vi "Local Endpoint B2.vi"() -> ()   [LabVIEW 2020]
uses:
  Communication/IP_Communication/typedefs/General Settings.ctl
  Communication/IP_Communication/typedefs/Endpoint Tag.ctl
  Communication/Local/Local.lvclass
  C:/Users/dihidalg/Documents/GitHub/lvoop_exercise1/Exercise Files/Communication/IP_Communication/IP_Communication.lvclass
  Communication/Network/Network.lvclass
  Communication/Packet/Packet.lvclass
  Communication/IP_Communication/IP_Communication.lvclass/IP_Communication.ctl
  Communication/Packet/Packet.lvclass/Packet.ctl
  Communication/IP_Communication/IP_Communication.lvclass
panel:
  in  "General Settings":T1={"Connection Name"="Local_Test", "Endpoint Tag"=enum."B"}
  in  "Local?":bool=TRUE
  in  "Stop VI":bool
  in  "Send Command":bool
  in  "Command ID":u16
  out "Command Rx":T3
  out "Timeout?":bool
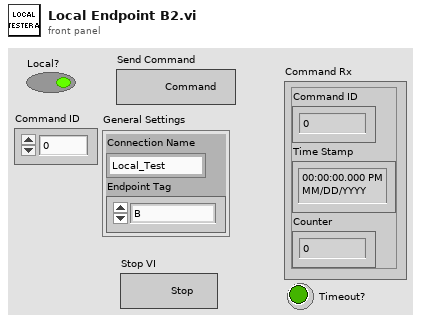
[diagram p1: front panel]
types:
  T1 = typedef "Communication Classes.lvlib/IP_Communication.lvclass/General Settings.ctl" = cluster{"Connection Name":string, "Endpoint Tag":T2}
  T2 = typedef "Communication Classes.lvlib/IP_Communication.lvclass/Endpoint Tag.ctl" = enum8{"A", "B"}
  T3 = cluster{"Command ID":u16, "Time Stamp":timestamp, "Counter":u16}
  T4 = cluster{"Command Out":cluster{"Command ID":u16, "Time Stamp":timestamp, "Counter":u16}, " Timeout?":bool}
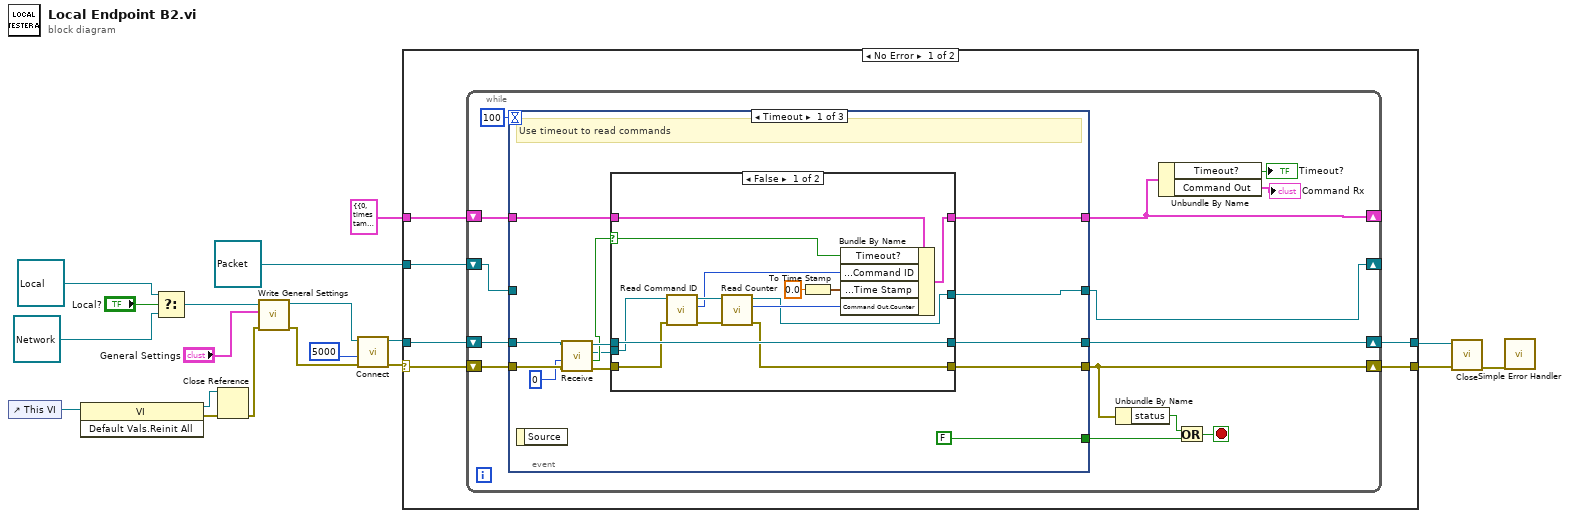
[diagram p0: block diagram]
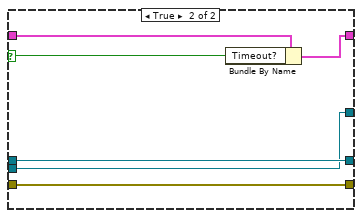
[diagram p2: hidden frame]
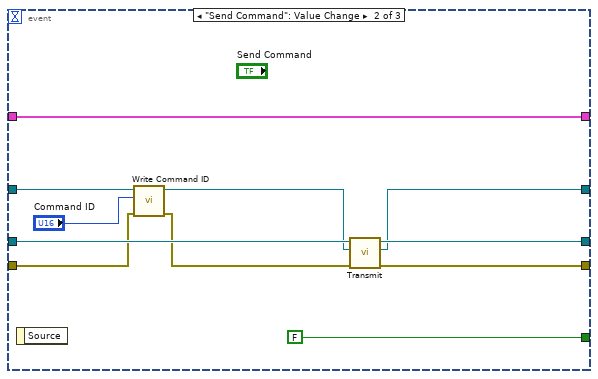
[diagram p3: hidden frame]
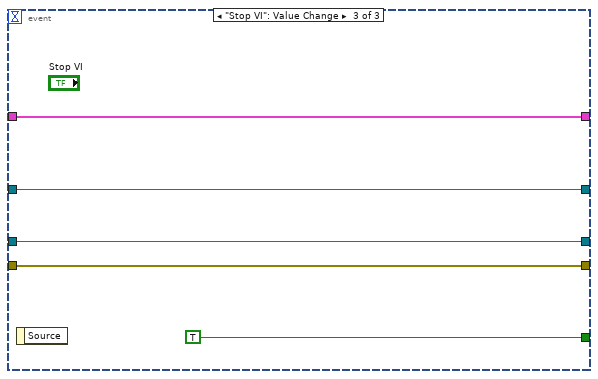
[diagram p4: hidden frame]
diagram:
  n1 = control-ref of="This VI"() -> (w19:refnum<vi>)
  n2 = invoke class="VI" method="Default Vals.Reinit All"(reference=w19) -> (reference out=w17:refnum<vi>, error out=w18:errorcluster)  [unwired: 2 in, 1 out]
  n3 = Select(t=refnum<class "Local.lvclass"> refnum ("Communication Classes.lvlib:Local.lvclass"), s="Local?", f=refnum<class "Network.lvclass"> refnum ("Communication Classes.lvlib:Network.lvclass")) -> (s? t:f=w5:refnum<class "IP_Communication.lvclass">)
  n4 = Close Reference(reference=w17, error in (no error)=w18) -> (error out=w3:errorcluster)
  n5 = call "Write General Settings.vi"("error in (no error)"=w3, "General Settings"="General Settings", "IP_Communication in"=w5) -> ("error out"=w2:errorcluster, "IP_Communication out"=w4:refnum<class "IP_Communication.lvclass">)  [unwired: 7 in]
  n6 = call-dynamic "Connect.vi"("error in (no error)"=w2, "timeout in ms (10000)"=5000 ("Timeout"), "Communication in"=w4) -> ("error out"=w13:errorcluster, "Communication out"=w12:refnum<class "IP_Communication.lvclass">)  [unwired: 7 in]
  n7 = case shown="No Error" w13 {
    selector: w13 -> [w21 w90]
    tunnel: [w23 w90] -> w10
    tunnel: [w22 w89] -> w8
    tunnel: w12 -> [w25 w89]
    tunnel: T4 {"Command Out"={"Command ID"=0, "Time Stamp"=timestamp(0 s since 1904-01-01), "Counter"=0}, " Timeout?"=FALSE} -> [w24 _]
    tunnel: refnum<class "Packet.lvclass"> refnum ("Communication Classes.lvlib:Packet.lvclass") -> [w20 _]
    frame No Error {
      n8 = while {
        shift-right: [w27] -> _
        shift-left: w24 -> [w38]
        shift-right: [w31] -> w22
        shift-left: w25 -> [w37]
        shift-right: [w35] -> w23
        shift-left: w21 -> [w36]
        shift-right: [w29] -> _
        shift-left: w20 -> [w30]
        stop <- w34 stop-if-true
        n9 = event shown="[0] Timeout" {
          selector: _ -> [_ _ _]
          dyn-events: _ -> [_ _ _]
          timeout: 100 -> [_ _ _]
          tunnel: w38 -> [w50 w83 w88]
          tunnel: [w49 w83 w88] -> w27
          tunnel: w37 -> [w48 w81 w84]
          tunnel: w36 -> [w47 w75 w87]
          tunnel: [w52 w78 w87] -> w35
          tunnel: [FALSE FALSE TRUE] -> w32
          tunnel: [w41 w76 w84] -> w31
          tunnel: w30 -> [_ w77 w85]
          tunnel: [w40 w73 w85] -> w29
          event Timeout {
            # "Use timeout to read commands"
            n10 = event-data() -> ()  [unwired: 1 in, 1 out]
            n11 = call-dynamic "Receive.vi"("error in (no error)"=w47, "timeout in ms (0)"=0 ("timeout in ms (-1)"), "Communication in"=w48) -> ("error out"=w43:errorcluster, "Timeout?"=w44:bool, "Packet Received"=w42:refnum<class "Packet.lvclass">, "Communication out"=w45:refnum<class "IP_Communication.lvclass">)  [unwired: 5 in]
            n12 = case shown="False" w44 {
              selector: w44 -> [w64 w69]
              tunnel: w43 -> [w58 w71]
              tunnel: w45 -> [w61 w72]
              tunnel: [w57 w71] -> w52
              tunnel: [w61 w72] -> w41
              tunnel: w42 -> [w56 w67]
              tunnel: w50 -> [w66 w70]
              tunnel: [w65 w68] -> w49
              tunnel: [w53 w67] -> w40
              frame False {
                n13 = call "Read Command ID.vi"("error in (no error)"=w58, "Packet in"=w56) -> ("error out"=w59:errorcluster, "Command ID"=w55:u16, "Packet out"=w60:refnum<class "Packet.lvclass">)  [unwired: 7 in]
                n14 = call "Read Counter.vi"("error in (no error)"=w59, "Packet in"=w60) -> ("error out"=w57:errorcluster, "Counter"=w54:u16, "Packet out"=w53:refnum<class "Packet.lvclass">)  [unwired: 7 in]
                n15 = To Time Stamp(1:0.0 ("number")) -> (0:w63:timestamp)
                n16 = Bundle By Name(cluster=w66, "Timeout?"=w64, "Command Out.Command ID"=w55, "Command Out.Time Stamp"=w63, "Command Out.Counter"=w54) -> (w65:T4)
              }
              frame True {
                n17 = Bundle By Name(cluster=w70, "Timeout?"=w69) -> (w68:T4)
              }
            }
          }
          event "Send Command": Value Change {
            n18 = event-data() -> ()  [unwired: 1 in, 1 out]
            n19 = call "Write Command ID.vi"("error in (no error)"=w75, "Command ID"="Command ID", "Packet in"=w77) -> ("error out"=w74:errorcluster, "Packet out"=w79:refnum<class "Packet.lvclass">)  [unwired: 7 in]
            n20 = call-dynamic "Transmit.vi"("error in (no error)"=w74, "Packet"=w79, "Communication In"=w81) -> ("error out"=w78:errorcluster, "Packet Sent"=w73:refnum<class "Packet.lvclass">, "Communication Out"=w76:refnum<class "IP_Communication.lvclass">)  [unwired: 5 in, 1 out]
          }
          event "Stop VI": Value Change {
            n21 = event-data() -> ()  [unwired: 1 in, 1 out]
          }
        }
        n22 = Unbundle By Name(w35) -> ("status"=w33:bool)
        n23 = Unbundle By Name(w27) -> ("Timeout?"=→"Timeout?":bool, "Command Out"=→"Command Rx":T3)
        n24 = Or(x=w33, y=w32) -> (x .or. y?=w34:bool)
      }
    }
    frame Error {
    }
  }
  n25 = call-dynamic "Close.vi"("error in (no error)"=w10, "Communication in"=w8) -> ("error out"=w9:errorcluster)  [unwired: 8 in, 1 out]
  n26 = call <vilib>:"Simple Error Handler.vi"("error in (no error)"=w9) -> ()  [unwired: 4 in, 5 out]
